vi "locker-Destroy.vi"(11 "Queue in":refnum<queue>) -> ()   [LabVIEW 2017, in "ObjectCacherAPI.lvlib"]
uses:
  ObjectCacherAPI.lvlib
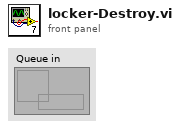
[diagram p1: front panel]
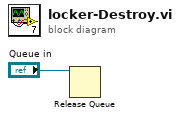
[diagram p0: block diagram]
diagram:
  n1 = Release Queue(queue="Queue in") -> ()  [unwired: 2 in, 3 out]
